vi "Swerve Drive.vi"(0 "X":dbl(slide)=-0.10236220472440945 scale=-1.0..1.0, 2 "Y":dbl(slide)=-0.07086614173228346 scale=1.0..-1.0, 5 "Z":dbl(knob)=0.13385826771653545 scale=1.0..-1.0, 6 "Rot. Point Y":dbl, 7 "Auto Controls":bool, 11 "Robot-Centric":bool, 12 "Rot. Point X":dbl) -> ()   [LabVIEW 2017]
uses:
  <vilib>/Rock Robotics/WPI/ThirdParty/Phoenix-LabVIEW/Motor Controller/Get/CTRE_Phoenix_MotorController_GetSelectedSensorData.vi
panel:
  out "Analog In-FL 4":dbl=535.0
  out "Sensor Position-FL 4":dbl=2.0
  in  "Ramp Rate-FL 4":dbl=60.0
  in  "I Zone-FL 4":dbl
  in  "F-FL 4":dbl=0.25
  in  "D-FL 4":dbl=0.5
  in  "I-FL 4":dbl=0.001
  in  "P-FL 4":dbl=4.0
  out "Analog In-FL 3":dbl=535.0
  out "Sensor Position-FL 3":dbl=2.0
  in  "Ramp Rate-FL 3":dbl=60.0
  in  "I Zone-FL 3":dbl
  in  "F-FL 3":dbl=0.25
  in  "D-FL 3":dbl=0.5
  in  "I-FL 3":dbl=0.001
  in  "P-FL 3":dbl=4.0
  out "Analog In-FL 2":dbl=535.0
  out "Sensor Position-FL 2":dbl=2.0
  in  "Ramp Rate-FL 2":dbl=60.0
  in  "I Zone-FL 2":dbl
  in  "F-FL 2":dbl=0.25
  in  "D-FL 2":dbl=0.5
  in  "I-FL 2":dbl=0.001
  in  "P-FL 2":dbl=4.0
  out "Analog In-FL":dbl=535.0
  out "Sensor Position-FL":dbl=2.0
  out "Robot Yaw":dbl=6.943359375
  in  "Ramp Rate-FL":dbl=60.0
  in  "I Zone-FL":dbl
  in  "F-FL":dbl=0.25
  in  "D-FL":dbl=0.5
  in  "I-FL":dbl=0.001
  in  "P-FL":dbl=4.0
  out "Rear Left\nAngle":dbl(knob) scale=-180.0..180.0 scale format="%#_3g"
  out "Rear Right\nAngle":dbl(knob) scale=-180.0..180.0 scale format="%#_3g"
  out "Front Right\nAngle":dbl(knob) scale=-180.0..180.0 scale format="%#_3g"
  out "Front Left\nAngle":dbl(knob) scale=-180.0..180.0 scale format="%#_3g"
  out "Rear Right\nCommand":dbl(knob) scale=-1.0..1.0 scale format="%#_3g"
  out "Rear Left\nCommand":dbl(knob) scale=-1.0..1.0 scale format="%#_3g"
  out "Front Right\nCommand":dbl(knob) scale=-1.0..1.0 scale format="%#_3g"
  out "Front Left\nCommand":dbl(knob) scale=-1.0..1.0 scale format="%#_3g"
  in  "Robot Length":dbl=21.625
  in  "Robot Width":dbl=20.0
  # "SWERVE DRIVE\nVersion 1.1\n12-25-2017\nTeam THRUST 1501"
  # "AndyMark\nSwerve Pod\nPID\nSoft Turns\nP=4\nI= 0.001\nD = 0.5\nFF = 0.25\nIZone = 0\nRamp = 40"
  # "AndyMark\nSwerve Pod\nPID\nAgressive\nP=0\nI= 0\nD = 0\nFF = 0\nIZone = 0\nRamp = 0"
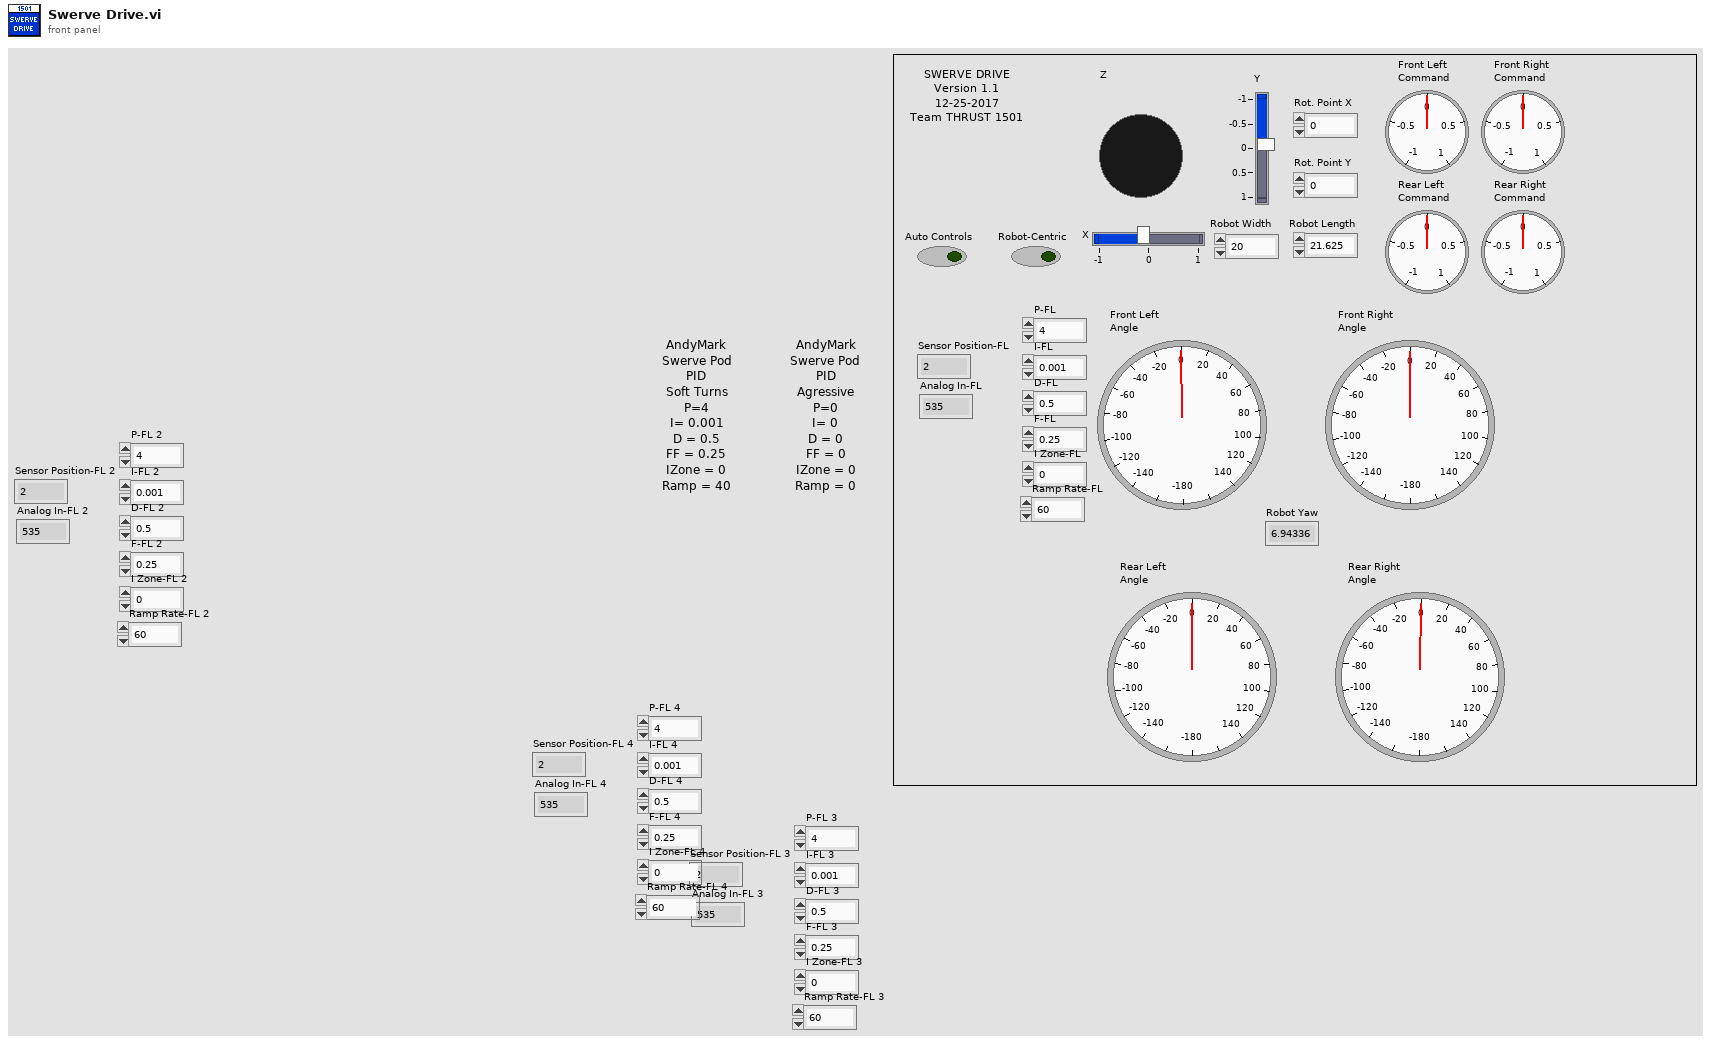
[diagram p1: front panel]
types:
  T1 = enum16{"Front Left", "Front Right", "Rear Right", "Rear Left"}
  T2 = typedef "WPI_MotorControlDeviceRef.ctl" = cluster{"DeviceStatus":errorcluster, "Type":T3, "PWM":cluster{"PWM Channel":T4, "DeadBand":T5}, "CAN":cluster{"Device Number":u8, "SetOutput VI Ref":variant, "GetOutput VI Ref":variant, "Enable VI Ref":variant, "Disable VI Ref":variant, "Data":variant}, "Invert":bool, "DIO PWM":cluster{"PWM \"Enable\" Channel":T4, "DIOChannel":T6, "PWM Rate":dbl}}
  T3 = typedef "WPI_MotorControlType.ctl" = enum16{"PWM", "CAN", "DIO PWM"}
  T4 = typedef "FPGA_DIOPWMChannel.ctl" = enum8{"PWM 0", "PWM 1", "PWM 2", "PWM 3", "PWM 4", "PWM 5", "PWM 6", "PWM 7", "PWM 8", "PWM 9", "PWM MXP 0", "PWM MXP 1", "PWM MXP 2", "PWM MXP 3", "PWM MXP 4", "PWM MXP 5", "PWM MXP 6", "PWM MXP 7", "PWM MXP 8", "PWM MXP 9", "Invalid"}
  T5 = typedef "WPI_PWMDeadband.ctl" = cluster{"Name":string, "maxPositivePwm":i32, "minPositivePwm":i32, "centerPwm":i32, "maxNegativePwm":i32, "minNegativePwm":i32, "angularRange":u16}
  T6 = typedef "FPGA_DIOChannel.ctl" = enum8{"DIO 0", "DIO 1", "DIO 2", "DIO 3", "DIO 4", "DIO 5", "DIO 6", "DIO 7", "DIO 8", "DIO 9", "DIO MXP 0", "DIO MXP 1", "DIO MXP 2", "DIO MXP 3", "DIO MXP 4", "DIO MXP 5", "DIO MXP 6", "DIO MXP 7", "DIO MXP 8", "DIO MXP 9", "DIO MXP 10", "DIO MXP 11", "DIO MXP 12", "DIO MXP 13", "DIO MXP 14", "DIO MXP 15", "SPI Port CS1", "SPI Port CS2", "SPI Port CS3", "SPI Port MISO", "SPI Port MOSI", "Invalid"}
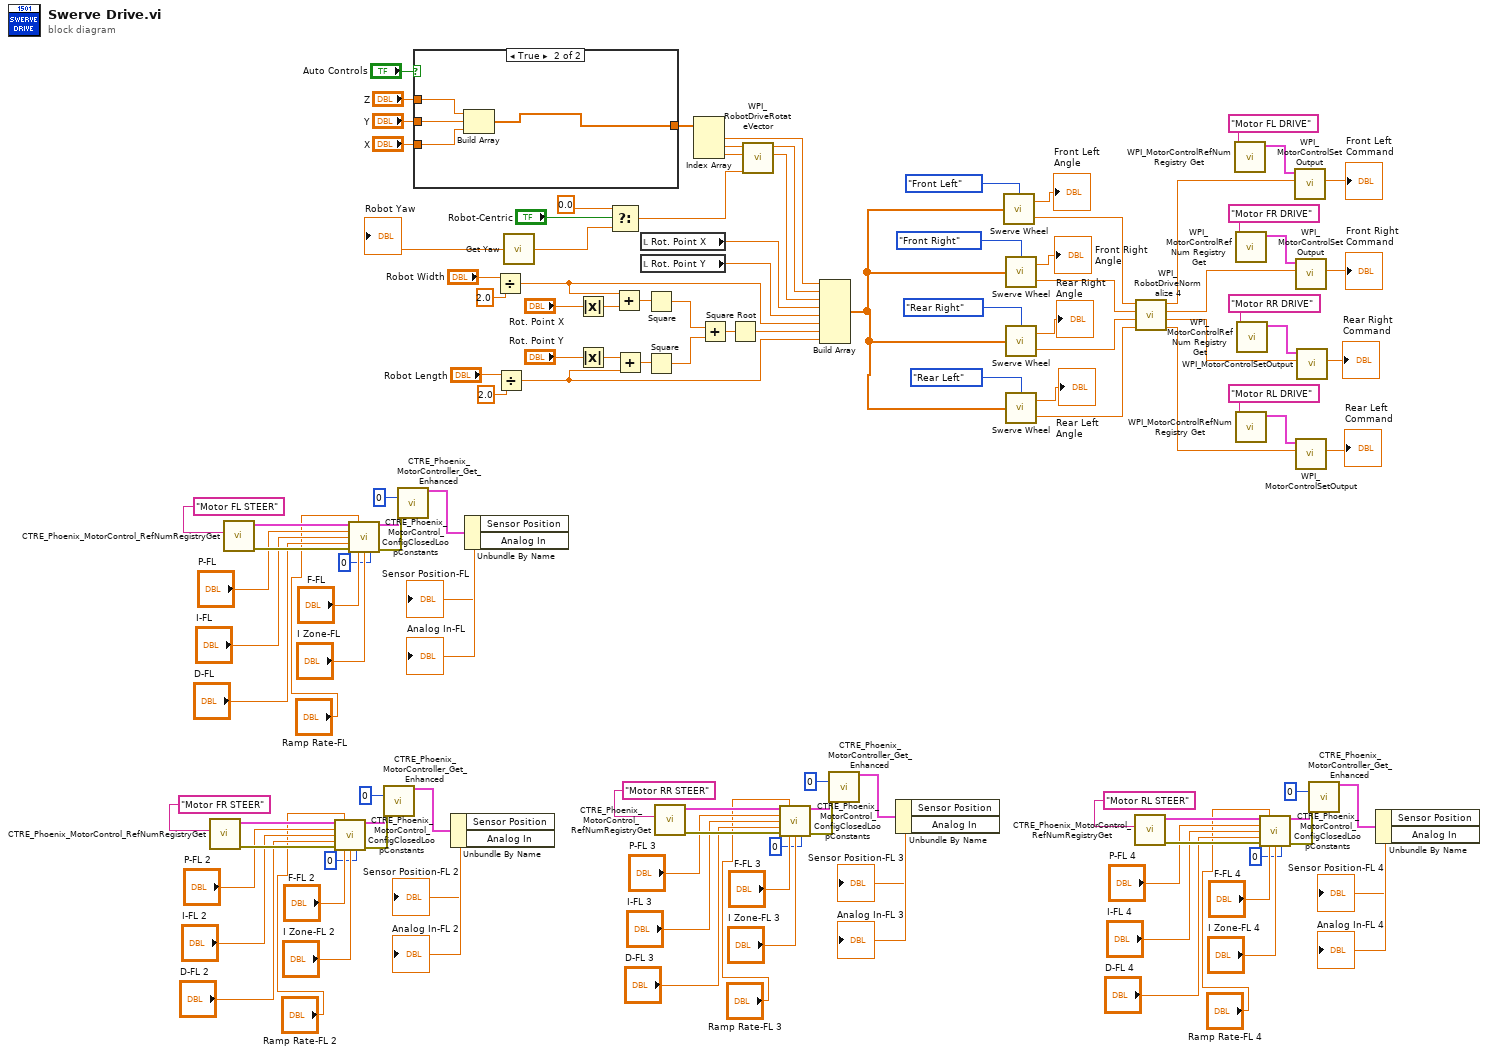
[diagram p0: block diagram]
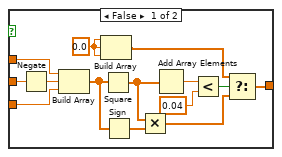
[diagram p2: hidden frame]
diagram:
  n1 = call <vilib>:"CTRE_Phoenix_MotorControl_RefNumRegistryGet.vi"("refnum name"="Motor FR STEER") -> ("error out"=w47:errorcluster, "PhoenixMotorControlDevRef"=w48:T2)  [unwired: 9 in]
  n2 = call <vilib>:"CTRE_Phoenix_MotorControl_RefNumRegistryGet.vi"("refnum name"="Motor FL STEER") -> ("error out"=w63:errorcluster, "PhoenixMotorControlDevRef"=w64:T2)  [unwired: 9 in]
  n3 = call <vilib>:"CTRE_Phoenix_MotorControl_ConfigClosedLoopConstants.vi"("PhoenixMotorControlDevRef"=w48, "slotIdx"="Ramp Rate-FL 2", "P"="P-FL 2", "I"="I-FL 2", "D"="D-FL 2", "error in (no error)"=w47, "F"="F-FL 2", "I Zone"="I Zone-FL 2", "timeoutMs"=0) -> ("PhoenixMotorControlDevRef"=w35:T2, "error out"=w36:errorcluster)  [unwired: 5 in]
  n4 = call <vilib>:"CTRE_Phoenix_MotorControl_ConfigClosedLoopConstants.vi"("PhoenixMotorControlDevRef"=w64, "slotIdx"="Ramp Rate-FL", "P"="P-FL", "I"="I-FL", "D"="D-FL", "error in (no error)"=w63, "F"="F-FL", "I Zone"="I Zone-FL", "timeoutMs"=0) -> ("PhoenixMotorControlDevRef"=w51:T2, "error out"=w52:errorcluster)  [unwired: 5 in]
  n5 = call-poly <vilib>:"CTRE_Phoenix_MotorController_Get_Enhanced.vi"("PhoenixMotorControlDevRef"=w35, "pidLoopIdx"=u32 0, "error in"=w36) -> ("PhoenixMotorControlDevRef"=w37:T2)  [unwired: 9 in, 3 out]
  n6 = call-poly <vilib>:"CTRE_Phoenix_MotorController_Get_Enhanced.vi"("PhoenixMotorControlDevRef"=w51, "pidLoopIdx"=u32 0, "error in"=w52) -> ("PhoenixMotorControlDevRef"=w53:T2)  [unwired: 9 in, 3 out]
  n7 = case shown="True" "Auto Controls" {
    tunnel: "Y" -> [w136 w142]
    tunnel: "X" -> [w130 w143]
    tunnel: "Z" -> [w126 w140]
    tunnel: [w127 w141] -> w87
    frame False {
      w134 = 0.0 ("element")
      n8 = Negate(x=w136) -> (-x=w129:dbl)
      n9 = Build Array(w126, w129, w130) -> (w133:dbl[])
      n10 = Build Array(w134, w134, w134) -> (w135:dbl[])
      n11 = Square(x=w133) -> (x^2=w131:dbl[])
      n12 = Sign(1:w133) -> (0:w132:dbl[])
      n13 = Multiply(x=w131, y=w132) -> (x*y=w128:dbl[])
      n14 = Add Array Elements(numeric array=w131) -> (sum=w139:dbl)
      n15 = Less?(x=w139, y=0.04 ("x")) -> (x < y?=w137:bool)
      n16 = Select(t=w135, s=w137, f=w128) -> (s? t:f=w127:dbl[])
    }
    frame True {
      n17 = Build Array(w140, w142, w143) -> (w141:dbl[])
    }
  }
  n18 = Unbundle By Name(w37) -> ("Sensor Position"=→"Sensor Position-FL 2":dbl, "Analog In"=→"Analog In-FL 2":dbl)
  n19 = Unbundle By Name(w53) -> ("Sensor Position"=→"Sensor Position-FL":dbl, "Analog In"=→"Analog In-FL":dbl)
  n20 = Divide(x="Robot Width", y=2.0) -> (x/y=w91:dbl)
  n21 = Divide(x="Robot Length", y=2.0) -> (x/y=w89:dbl)
  n22 = call "Get Yaw.vi"() -> ("Angle"=w65:dbl)  [unwired: 1 in]
  "Robot Yaw" <- w65
  n23 = Absolute Value(x="Rot. Point X") -> (abs(x)=w109:dbl)
  n24 = Absolute Value(x="Rot. Point Y") -> (abs(x)=w107:dbl)
  n25 = Select(t=0.0, s="Robot-Centric", f=w65) -> (s? t:f=w82:dbl)
  n26 = Add(x=w91, y=w109) -> (x+y=w108:dbl)
  n27 = Add(x=w107, y=w89) -> (x+y=w106:dbl)
  n28 = local read "Rot. Point X"() -> (w93:dbl)
  n29 = local read "Rot. Point Y"() -> (w92:dbl)
  n30 = Square(x=w108) -> (x^2=w104:dbl)
  n31 = Square(x=w106) -> (x^2=w105:dbl)
  n32 = call <vilib>:"CTRE_Phoenix_MotorControl_RefNumRegistryGet.vi"("refnum name"="Motor RR STEER") -> ("error out"=w31:errorcluster, "PhoenixMotorControlDevRef"=w32:T2)  [unwired: 9 in]
  n33 = Index Array(array=w87) -> (element #1=w81:dbl, element #2=w88:dbl, element #3=w96:dbl)  [unwired: 3 in]
  n34 = Add(x=w104, y=w105) -> (x+y=w103:dbl)
  n35 = Square Root(x=w103) -> (sqrt(x)=w90:dbl)
  n36 = call <vilib>:"WPI_RobotDriveRotateVector.vi"("Angle"=w82, "X"=w96, "Y"=w88) -> ("X'"=w85:dbl, "Y'"=w80:dbl)  [unwired: 7 out]
  n37 = call <vilib>:"CTRE_Phoenix_MotorControl_ConfigClosedLoopConstants.vi"("PhoenixMotorControlDevRef"=w32, "slotIdx"="Ramp Rate-FL 3", "P"="P-FL 3", "I"="I-FL 3", "D"="D-FL 3", "error in (no error)"=w31, "F"="F-FL 3", "I Zone"="I Zone-FL 3", "timeoutMs"=0) -> ("PhoenixMotorControlDevRef"=w19:T2, "error out"=w20:errorcluster)  [unwired: 5 in]
  n38 = Build Array(w81, w80, w85, w93, w92, w91, w90, w89) -> (w86:dbl[])
  n39 = call-poly <vilib>:"CTRE_Phoenix_MotorController_Get_Enhanced.vi"("PhoenixMotorControlDevRef"=w19, "pidLoopIdx"=u32 0, "error in"=w20) -> ("PhoenixMotorControlDevRef"=w21:T2)  [unwired: 9 in, 3 out]
  n40 = Unbundle By Name(w21) -> ("Sensor Position"=→"Sensor Position-FL 3":dbl, "Analog In"=→"Analog In-FL 3":dbl)
  n41 = call "Swerve Wheel.vi"("Wheel"=T1."Front Left", "Inputs"=w86) -> ("Speed"=w125:dbl, "Angle"=→"Front Left\nAngle":dbl)  [unwired: 2 in]
  n42 = call "Swerve Wheel.vi"("Wheel"=T1."Front Right", "Inputs"=w86) -> ("Speed"=w124:dbl, "Angle"=→"Front Right\nAngle":dbl)  [unwired: 2 in]
  n43 = call "Swerve Wheel.vi"("Wheel"=T1."Rear Right", "Inputs"=w86) -> ("Speed"=w123:dbl, "Angle"=→"Rear Right\nAngle":dbl)  [unwired: 2 in]
  n44 = call "Swerve Wheel.vi"("Wheel"=T1."Rear Left", "Inputs"=w86) -> ("Speed"=w122:dbl, "Angle"=→"Rear Left\nAngle":dbl)  [unwired: 2 in]
  n45 = call <vilib>:"CTRE_Phoenix_MotorControl_RefNumRegistryGet.vi"("refnum name"="Motor RL STEER") -> ("error out"=w15:errorcluster, "PhoenixMotorControlDevRef"=w16:T2)  [unwired: 9 in]
  n46 = call <vilib>:"WPI_RobotDriveNormalize 4.vi"("D"=w122, "C"=w123, "B"=w124, "A"=w125) -> ("D'"=w111:dbl, "C'"=w112:dbl, "B'"=w113:dbl, "A'"=w74:dbl)
  n47 = call <vilib>:"WPI_MotorControlRefNum Registry Get.vi"("refnum name"="Motor FL DRIVE") -> ("MotorControlDevRef"=w121:T2)  [unwired: 9 in, 1 out]
  n48 = call <vilib>:"WPI_MotorControlRefNum Registry Get.vi"("refnum name"="Motor FR DRIVE") -> ("MotorControlDevRef"=w118:T2)  [unwired: 9 in, 1 out]
  n49 = call <vilib>:"WPI_MotorControlRefNum Registry Get.vi"("refnum name"="Motor RL DRIVE") -> ("MotorControlDevRef"=w114:T2)  [unwired: 9 in, 1 out]
  n50 = call <vilib>:"WPI_MotorControlRefNum Registry Get.vi"("refnum name"="Motor RR DRIVE") -> ("MotorControlDevRef"=w117:T2)  [unwired: 9 in, 1 out]
  n51 = call <vilib>:"CTRE_Phoenix_MotorControl_ConfigClosedLoopConstants.vi"("PhoenixMotorControlDevRef"=w16, "slotIdx"="Ramp Rate-FL 4", "P"="P-FL 4", "I"="I-FL 4", "D"="D-FL 4", "error in (no error)"=w15, "F"="F-FL 4", "I Zone"="I Zone-FL 4", "timeoutMs"=0) -> ("PhoenixMotorControlDevRef"=w3:T2, "error out"=w4:errorcluster)  [unwired: 5 in]
  n52 = call <vilib>:"WPI_MotorControlSetOutput.vi"("Output"=w74, "MotorControlDevRef"=w121) -> ("Motor Output"=→"Front Left\nCommand":dbl)  [unwired: 7 in, 2 out]
  n53 = call <vilib>:"WPI_MotorControlSetOutput.vi"("Output"=w113, "MotorControlDevRef"=w118) -> ("Motor Output"=→"Front Right\nCommand":dbl)  [unwired: 7 in, 2 out]
  n54 = call <vilib>:"WPI_MotorControlSetOutput.vi"("Output"=w111, "MotorControlDevRef"=w114) -> ("Motor Output"=→"Rear Left\nCommand":dbl)  [unwired: 7 in, 2 out]
  n55 = call <vilib>:"WPI_MotorControlSetOutput.vi"("Output"=w112, "MotorControlDevRef"=w117) -> ("Motor Output"=→"Rear Right\nCommand":dbl)  [unwired: 7 in, 2 out]
  n56 = call-poly <vilib>:"CTRE_Phoenix_MotorController_Get_Enhanced.vi"("PhoenixMotorControlDevRef"=w3, "pidLoopIdx"=u32 0, "error in"=w4) -> ("PhoenixMotorControlDevRef"=w5:T2)  [unwired: 9 in, 3 out]
  n57 = Unbundle By Name(w5) -> ("Sensor Position"=→"Sensor Position-FL 4":dbl, "Analog In"=→"Analog In-FL 4":dbl)
